vi "PyroReadConf.vi"(8 "error in":errorcluster, 10 "PyroClusterIn":T1={"COM"=0, "Good"=FALSE, "Address"=0, "Emissivity"=0.0, "T95"=21, "Temp(K)"=0.0, "Time"=timestamp(0 s since 1904-01-01), "Laser"=FALSE} {"T95" items=["min/off"=0, "1ms"=10, "2ms"=11, "5ms"=12, "10ms"=13, "20ms"=14, "50ms"=15, "100ms"=16, "200ms"=17, "500ms"=18, "1s"=19, "2s"=20, "5s"=21, "10s"=22, "20s"=23, "50s"=24, "100s"=25]}, 11 "StructIn":T3) -> (0 "error out":errorcluster, 2 "PyroClusterOut":T1={"COM"=0, "Good"=FALSE, "Address"=0, "Emissivity"=0.0, "T95"=21, "Temp(K)"=0.0, "Time"=timestamp(0 s since 1904-01-01), "Laser"=FALSE} {"T95" items=["min/off"=0, "1ms"=10, "2ms"=11, "5ms"=12, "10ms"=13, "20ms"=14, "50ms"=15, "100ms"=16, "200ms"=17, "500ms"=18, "1s"=19, "2s"=20, "5s"=21, "10s"=22, "20s"=23, "50s"=24, "100s"=25]}, 3 "StructOut":T3)   [LabVIEW 2021]
uses:
  DIAS_Pyrometer/VIs/Server/PyrospotDat.ctl
  DIAS_Pyrometer/VIs/Server/TimeResp.ctl
  Library/TerminalDef.ctl
  <vilib>/Utility/config.llb/Config Data RefNum.ctl
  Library/LibDan.lvlib
  DIAS_Pyrometer/DIAS_Pyrometer.lvlib
  <vilib>/Utility/config.llb/NI_LVConfig.lvlib
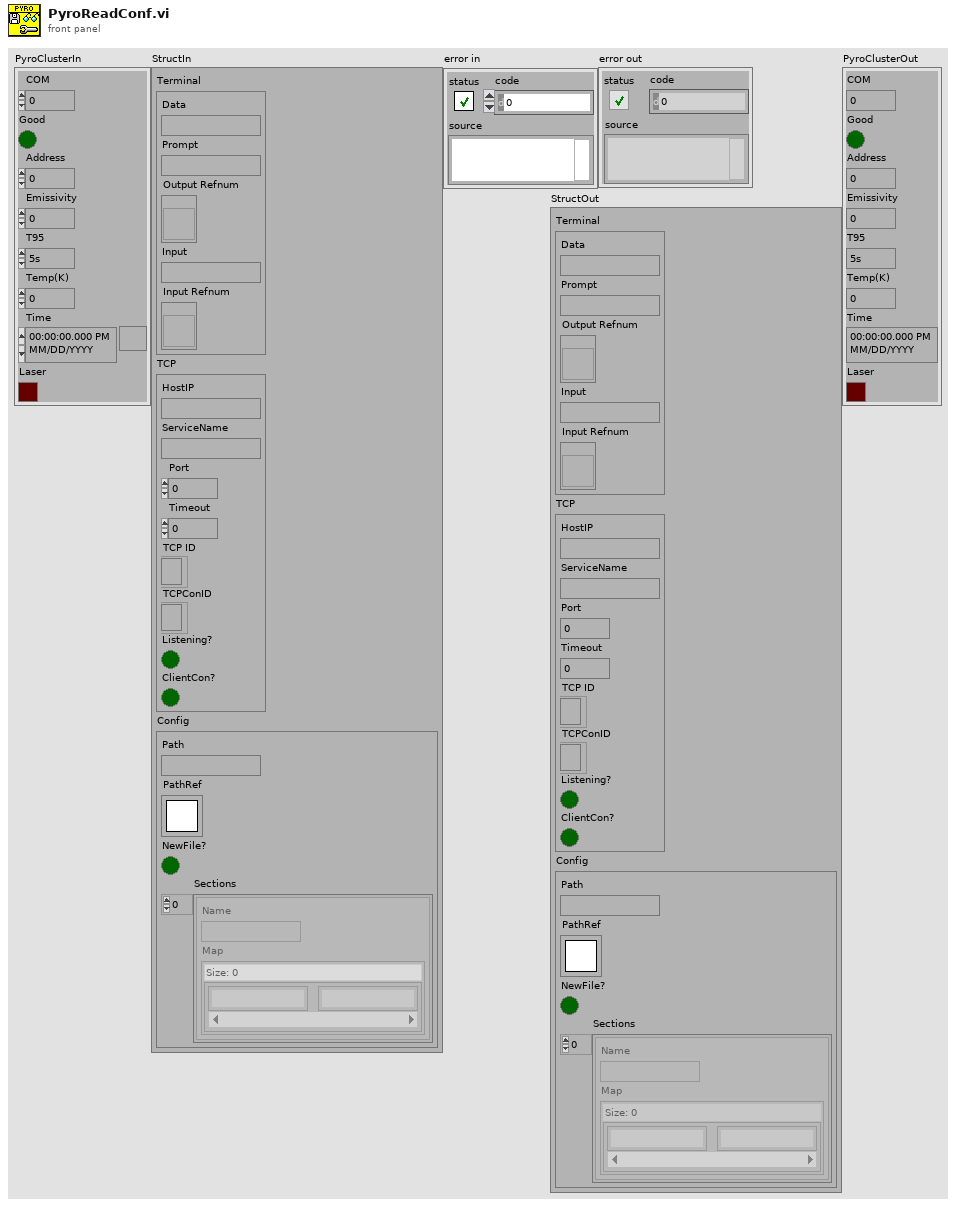
[diagram p1: front panel]
types:
  T1 = typedef "DIAS_Pyrometer.lvlib/PyrospotDat.ctl" = cluster{"COM":u16, "Good":bool, "Address":i32, "Emissivity":sgl, "T95":T2, "Temp(K)":dbl, "Time":timestamp, "Laser":bool}
  T2 = typedef "DIAS_Pyrometer.lvlib/TimeResp.ctl" = u16
  T3 = typedef "LibDan.lvlib/TerminalDef.ctl" = cluster{"Terminal":cluster{"Data":string, "Prompt":string, "Output Refnum":refnum<vi>, "Input":string, "Input Refnum":refnum<vi>}, "TCP":cluster{"HostIP":string, "ServiceName":string, "Port":u16, "Timeout":i32, "TCP ID":refnum<k5>, "TCPConID":refnum<k5>, "Listening?":bool, "ClientCon?":bool}, "Config":cluster{"Path":path, "PathRef":T4, "NewFile?":bool, "Sections":cluster{"Name":string, "Map":map{string, string}}[]}}
  T4 = typedef "NI_LVConfig.lvlib/Config Data RefNum.ctl" = refnum<k1>
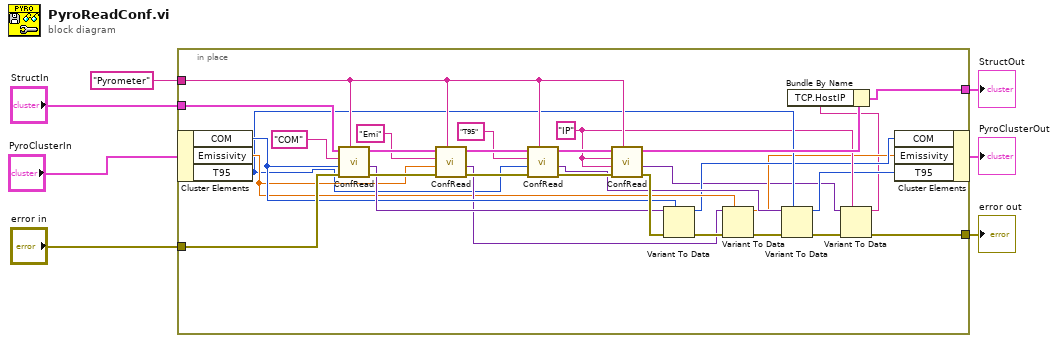
[diagram p0: block diagram]
diagram:
  n1 = in-place {
    in-place-border: "StructIn" -> [w26]
    in-place-border: "Pyrometer" ("Section") -> [w29]
    in-place-border: "error in" -> [w36]
    in-place-border: [w27] -> w2
    in-place-border: [w9] -> w3
    w14 = "IP" ("key")
    n2 = in-place-cluster #1("PyroClusterIn") -> ("COM"=w22:u16, "Emissivity"=w19:sgl, "T95"=w16:T2)
    n3 = call "ConfRead.vi"("Section"=w29, "error in"=w36, "type"=w22, "key"="COM", "StructIn"=w26) -> ("error out"=w25:errorcluster, "value"=w23:variant, "StructOut"=w38:T3)  [unwired: 4 in]
    n4 = call "ConfRead.vi"("Section"=w29, "error in"=w25, "type"=w19, "key"="Emi", "StructIn"=w38) -> ("error out"=w34:errorcluster, "value"=w20:variant, "StructOut"=w35:T3)  [unwired: 4 in]
    n5 = call "ConfRead.vi"("Section"=w29, "error in"=w34, "type"=w16, "key"="T95", "StructIn"=w35) -> ("error out"=w30:errorcluster, "value"=w17:variant, "StructOut"=w31:T3)  [unwired: 4 in]
    n6 = call "ConfRead.vi"("Section"=w29, "error in"=w30, "type"=w14, "key"=w14, "StructIn"=w31) -> ("error out"=w24:errorcluster, "value"=w8:variant, "StructOut"=w28:T3)  [unwired: 4 in]
    n7 = Variant To Data(error in=w24, type=w22, Variant=w23) -> (data=w13:u16, error out=w21:errorcluster)
    n8 = Variant To Data(error in=w21, type=w19, Variant=w20) -> (data=w12:sgl, error out=w18:errorcluster)
    n9 = Variant To Data(error in=w18, type=w16, Variant=w17) -> (data=w11:T2, error out=w15:errorcluster)
    n10 = Variant To Data(error in=w15, type=w14, Variant=w8) -> (data=w10:string, error out=w9:errorcluster)
    n11 = Bundle By Name(cluster=w28, "TCP.HostIP"=w10) -> (w27:T3)
    n12 = in-place-cluster #1("COM"=w13, "Emissivity"=w12, "T95"=w11) -> (→"PyroClusterOut":T1)
  }
  "error out" <- w3
  "StructOut" <- w2
